vi "_02_Create a S-VI.vi"(7 "Enum":enum16{"Read Data", "Write Data"}(ring), 8 "error in (no error)":errorcluster, 11 "i/p":dbl) -> (0 "error out":errorcluster, 3 "o/p":dbl)   [LabVIEW 2020]
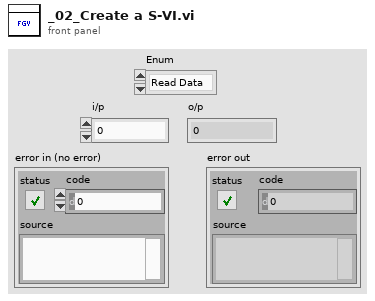
[diagram p1: front panel]
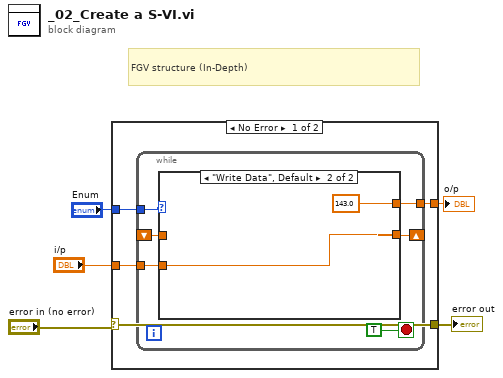
[diagram p0: block diagram]
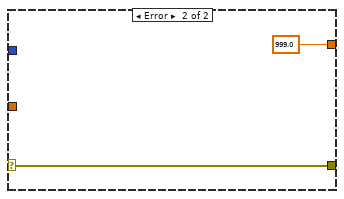
[diagram p3: hidden frame]
diagram:
  # "FGV structure (In-Depth)"
  n1 = case shown="No Error" "error in (no error)" {
    selector: "error in (no error)" -> [w6 w20]
    tunnel: [w6 w20] -> w2
    tunnel: "Enum" -> [w9 _]
    tunnel: "i/p" -> [w8 _]
    tunnel: [w7 999.0 ("i/p")] -> w5
    frame No Error {
      n2 = while {
        tunnel: w9 -> [w15]
        shift-right: [w13] -> _
        shift-left: _ -> [w12]
        tunnel: w8 -> [w14]
        tunnel: [w11] -> w7
        stop <- TRUE stop-if-true
        n3 = case shown="\"Write Data\", Default" w15 {
          tunnel: w14 -> [_ w18]
          tunnel: [w16 w18] -> w13
          tunnel: w12 -> [w16 _]
          tunnel: [w16 143.0 ("i/p")] -> w11
          frame "Read Data" {
          }
          frame "Write Data", Default {
          }
        }
      }
    }
    frame Error {
    }
  }
  "o/p" <- w5
  "error out" <- w2
